vi "Read Device.vi"(8 "error in (no error)":errorcluster, 11 "ATS9350 in":refnum<class "ATS9350.lvclass">) -> (0 "error out":errorcluster, 2 "Device":i32, 3 "ATS9350 out":refnum<class "ATS9350.lvclass">)   [LabVIEW 2014, in "ATS9350.lvclass"]
uses:
  ATS9350.lvclass
  ATS9350.lvclass/ATS9350.ctl
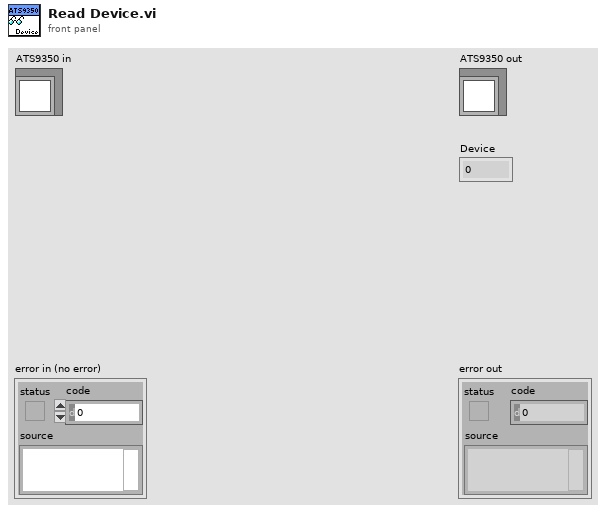
[diagram p1: front panel]
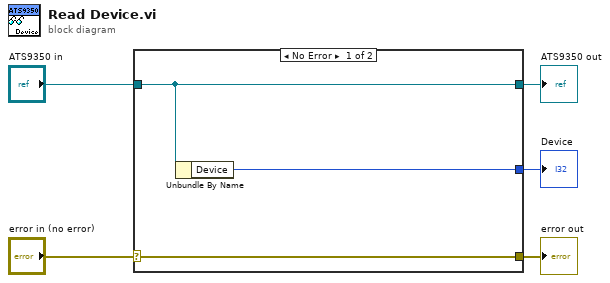
[diagram p0: block diagram]
diagram:
  n1 = case shown="No Error" "error in (no error)" {
    selector: "error in (no error)" -> [w8 w9]
    tunnel: [w8 w9] -> w4
    tunnel: [w7 w10] -> w2
    tunnel: "ATS9350 in" -> [w7 w10]
    tunnel: [w6 _] -> w1
    frame No Error {
      n2 = Unbundle By Name(w7) -> ("Device"=w6:i32)
    }
    frame Error {
    }
  }
  "error out" <- w4
  "ATS9350 out" <- w2
  "Device" <- w1
